vi "SP_OEE_2_test.vi"() -> ()   [LabVIEW 2017]
uses:
  <vilib>/addons/database/Connection.llb/DB Tools Open Connec (Path).vi
  <vilib>/addons/database/_DB Variant To Data/Database Variant To Data.xnode
  <vilib>/addons/database/NI_Database_API.lvlib
panel:
  in  "Left Button":bool
  in  "Report Button":bool
  out "Array":string[][](array[string])
  out "OEE":dbl format="%#_4g"
  out "IDEAL CYCLE TIME":i32
  out "CAPACITY":dbl
  out "AVAILABLILITY TIME(MIN)":i32
  out "PERFORMANCE":dbl format="%#_4g"
  out "QUALITY":dbl format="%#_4g"
  out "Production count":i32
  out "transposed array":string[][](array[string])
  out "CYCLE TIME":string[](array[string])
  out "ACTUAL PROD TIME":string[](array[string])
  out "?":string[][](array[string])
  out "error out":errorcluster
  in  "wise":string(combo)
  out "Date Count":string[](array[string])
  out "Sorted Date":string[](array[string])
  out "ALL DATE":string[](array[string])
  in  "error in (no error)":errorcluster
  in  "Download":bool
  in  "Shift":string(combo)
  in  "Tab Control":enum32{"Statistical", "Graphical"}(tab)
  out "Table":string[][](table)
  out "Table 2":string[][](table)
  out "Run-Time Status":cluster{"Array 2":timestamp[], dbl[]}(graph)
  in  "Select Station":string(combo)
  in  "To Date":timestamp format="%<%Y-%m-%d>T"
  in  "Form Date":timestamp format="%<%Y-%m-%d>T"
  in  "Select Stakeholder":string(combo)
  # "OEE REPORT"
  # "%"
  # "Date"
  # "Safety"
  # "Logistic"
  # "Maintenance"
  # "Quality"
  # "Production"
  # "Total"
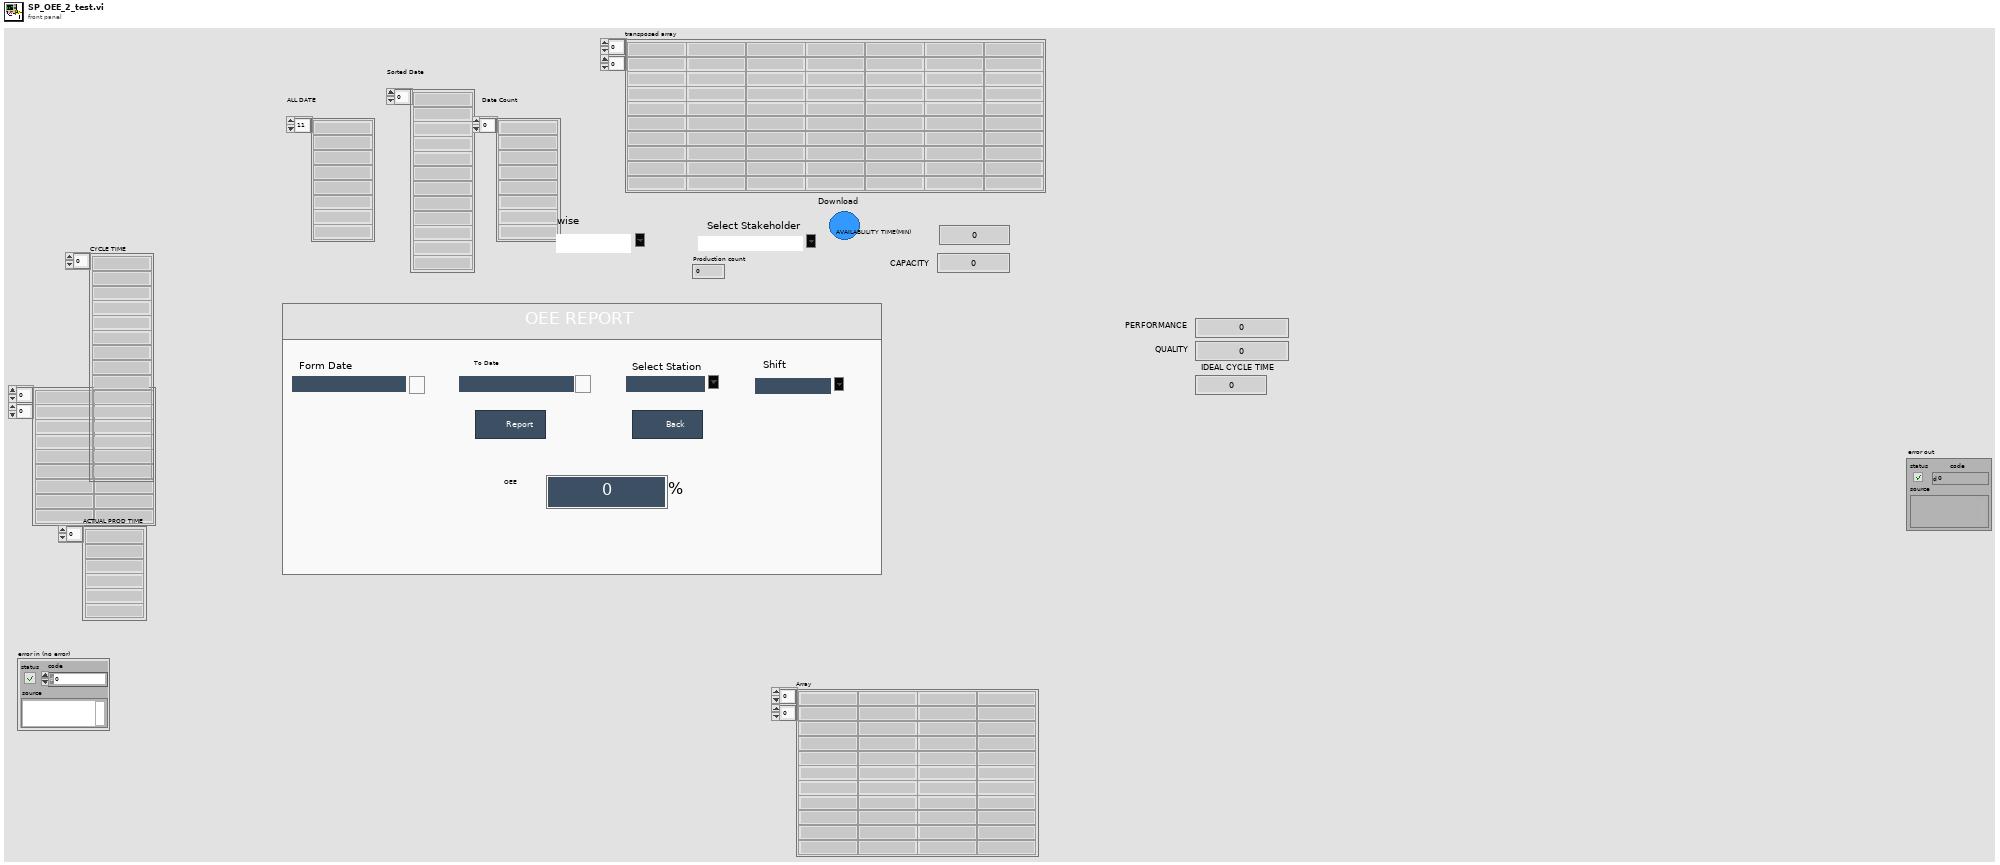
[diagram p1: front panel]
types:
  T1 = typedef "LVDateTimeRec.ctl" = cluster{"fractional second":dbl, "second":i32, "minute":i32, "hour":i32, "day of month":i32, "month":i32, "year":i32, "day of week":i32, "day of year":i32, "DST":i32}
  T2 = typedef "NI_Database_API.lvlib/Conn ObjectReference.ctl" = refnum<k1>
  T3 = enum32{"invalid app kind", "Development System", "Run Time System", "Student Edition", "Embedded LabVIEW", "Evaluation", "Custom"}
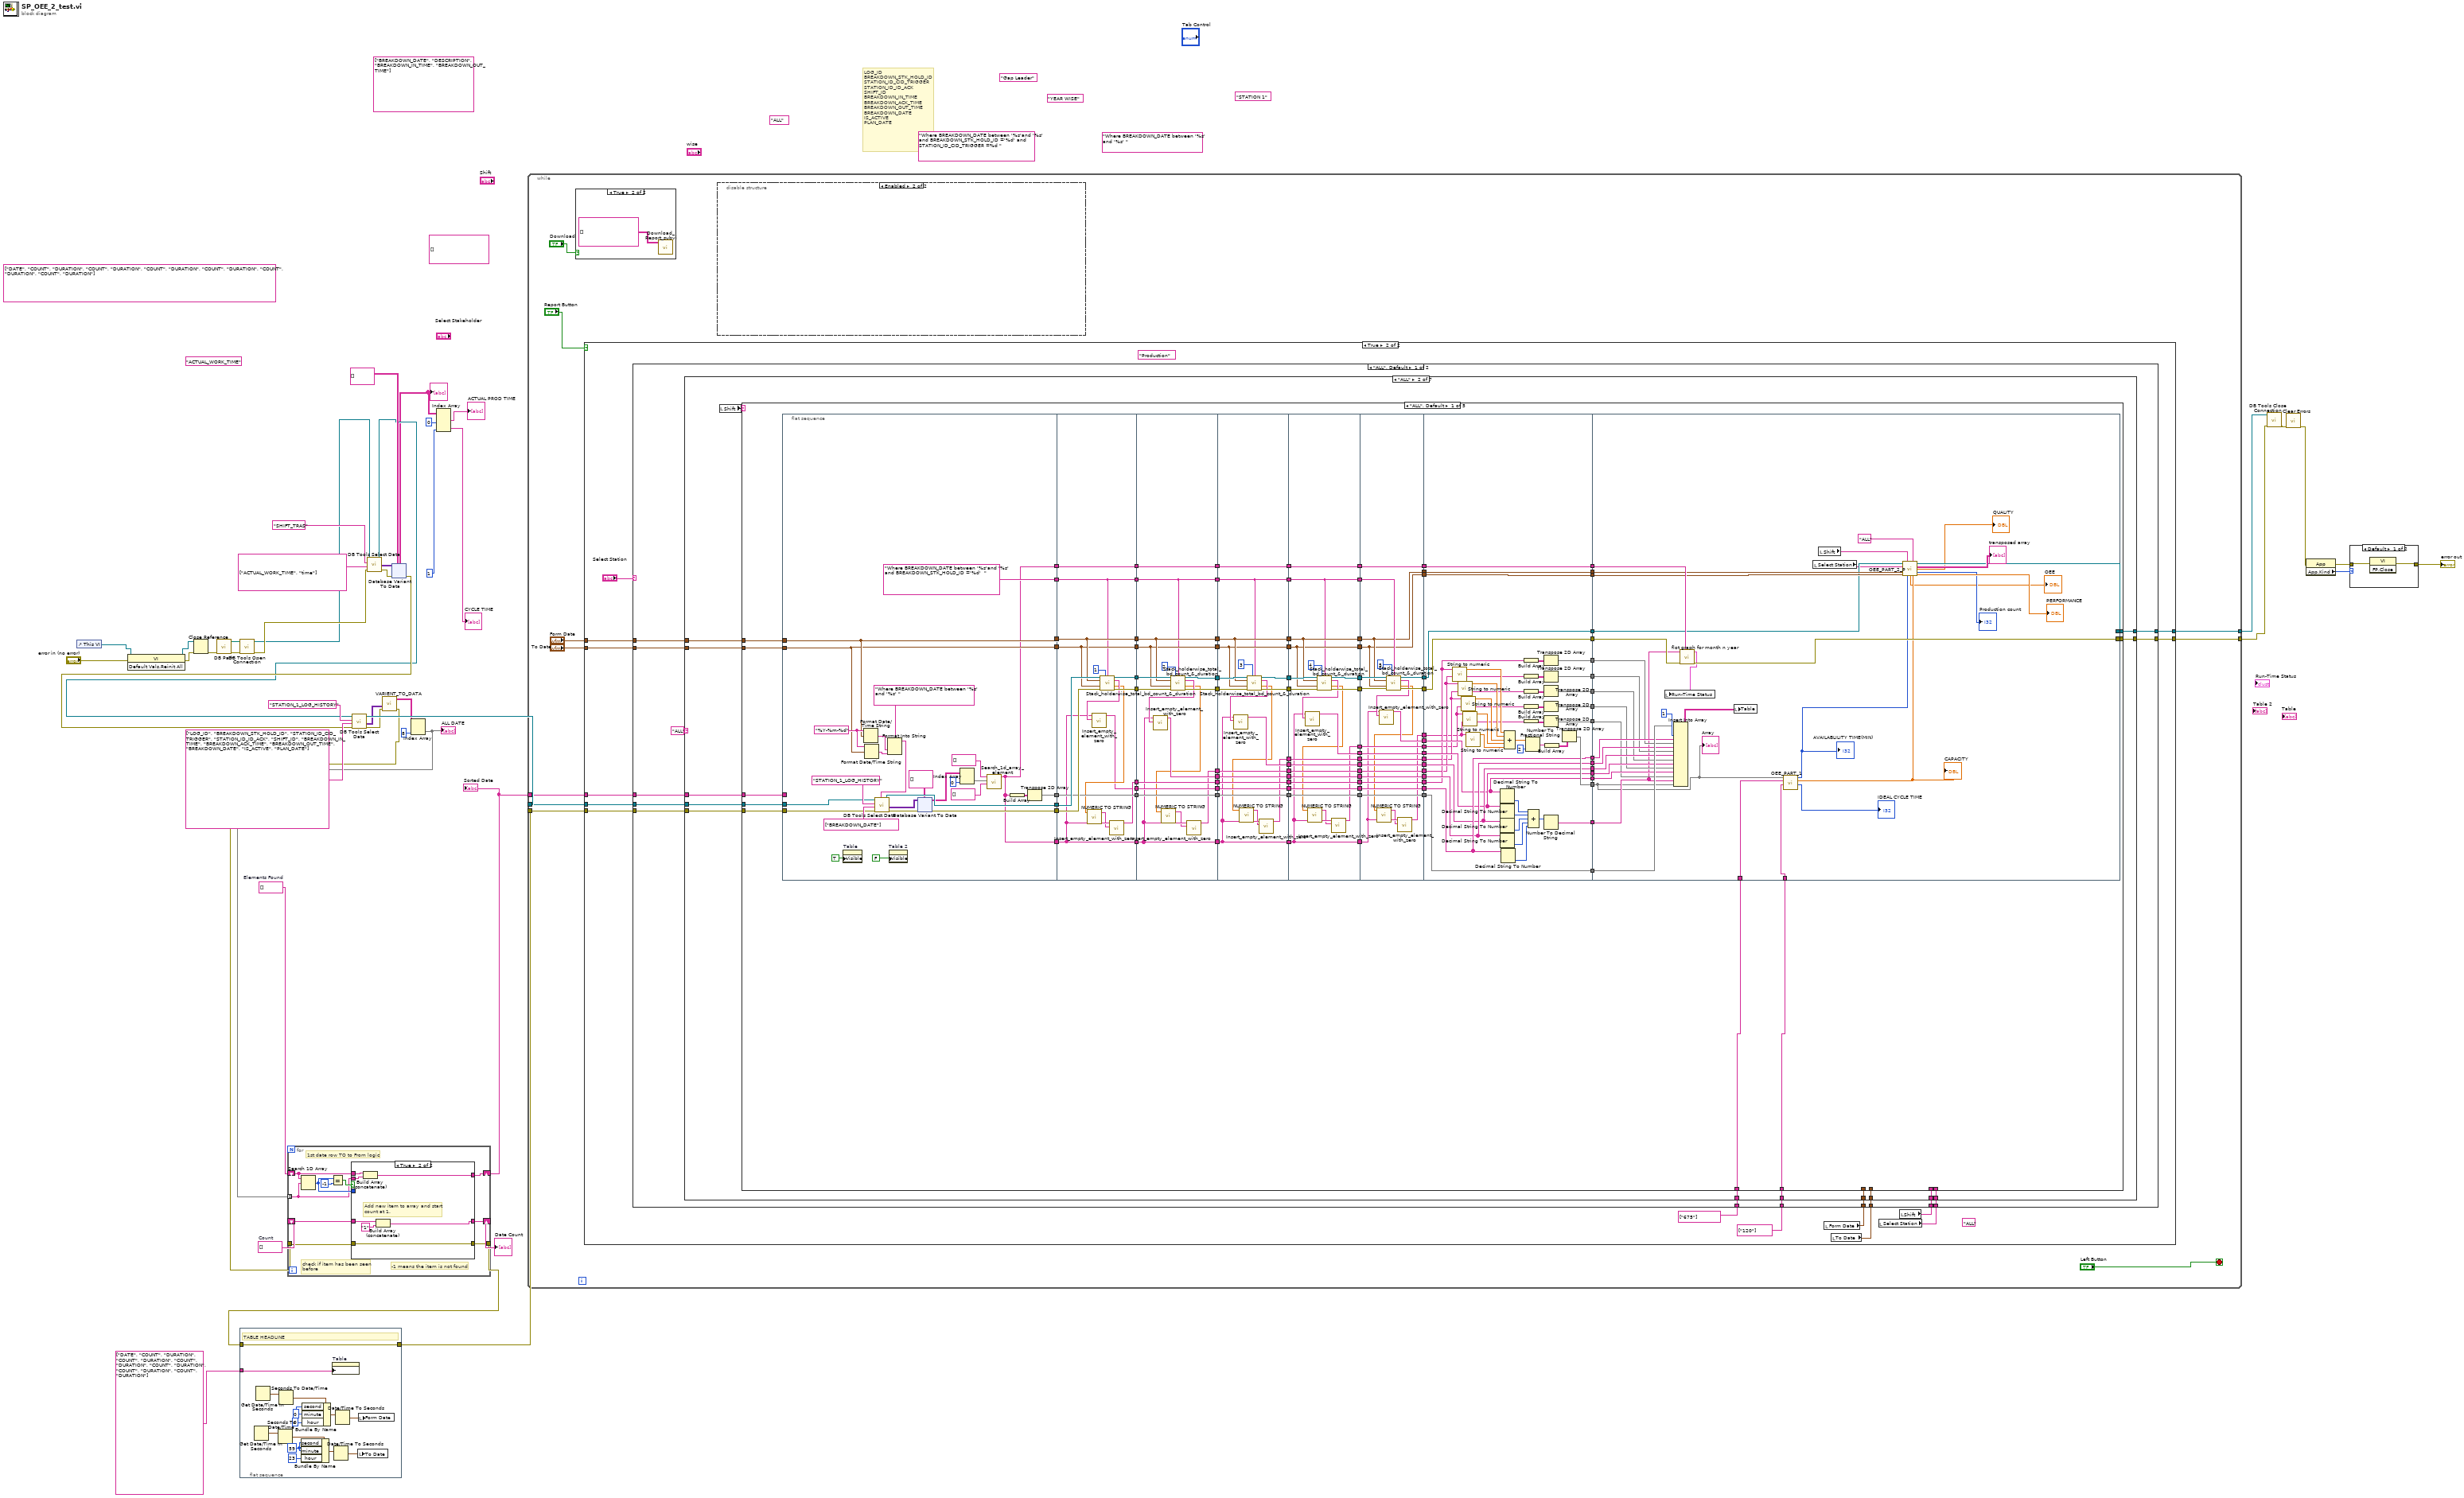
[diagram p0: block diagram]
diagram:
  (unwired) string[][] [] ("Column Header Strings[]")
  (unwired) string[][] [["DATE", "COUNT", "DURATION", "COUNT", "DURATION", "COUNT", "DURATION", "COUNT", "DURATION", "COUNT", "DURATION", "COUNT", "DURATION"]] ("Column Header Strings[]")
  (unwired) "ACTUAL_WORK_TIME" ("String")
  (unwired) "Where BREAKDOWN_DATE between '%s' and '%s' "
  (unwired) "Where BREAKDOWN_DATE between '%s'and '%s' and BREAKDOWN_STK_HOLD_ID ='%d' and STATION_ID_CID_TRIGGER =%d "
  (unwired) "ALL" ("Shift")
  (unwired) "STATION 1" ("Select Station")
  (unwired) "Gap Leader" ("Select Stakeholder")
  (unwired) string[] ["BREAKDOWN_DATE", "DESCRIPTION", "BREAKDOWN_IN_TIME", "BREAKDOWN_OUT_TIME"]
  (unwired) "YEAR WISE" ("wise")
  w34 = string[] []  # Count
  w35 = string[] []  # Elements Found
  # "LOG_ID\nBREAKDOWN_STK_HOLD_ID\nSTATION_ID_CID_TRIGGER\nSTATION_ID_ID_ACK\nSHIFT_ID\nBREAKDOWN_IN_TIME\nBREAKDOWN_ACK_TIME\nBREAKDOWN_OUT_TIME\nBREAKDOWN_DATE\nIS_ACTIVE\nPLAN_DATE"
  n1 = control-ref of="This VI"() -> (w44:refnum<vi>)
  n2 = invoke class="VI" method="Default Vals.Reinit All"(reference=w44, error in="error in (no error)") -> (reference out=w42:refnum<vi>, error out=w43:errorcluster)  [unwired: 1 in, 1 out]
  n3 = Close Reference(reference=w42, error in (no error)=w43) -> (error out=w41:errorcluster)
  n4 = call "DB Path.vi"("error in"=w41) -> ("error out"=w40:errorcluster, "DB Path"=w39:path)  [unwired: 9 in]
  n5 = flat-sequence {
    tunnel: [w58] -> w27
    tunnel: w30 -> [w58]
    tunnel: string[] ["DATE", "COUNT", "DURATION", "COUNT", "DURATION", "COUNT", "DURATION", "COUNT", "DURATION", "COUNT", "DURATION", "COUNT", "DURATION"] ("Column Header Strings[]") -> [w45]
    frame #0 {
      w48 = 59 ("second")
      w54 = 0 ("second")
      # "TABLE HEADLINE"
      n6 = Get Date/Time In Seconds() -> (seconds since 1Jan1904=w51:timestamp)
      n7 = Get Date/Time In Seconds() -> (seconds since 1Jan1904=w55:timestamp)
      n8 = Seconds To Date/Time(time stamp (now)=w51) -> (date time rec=w50:T1)  [unwired: 1 in]
      n9 = Seconds To Date/Time(time stamp (now)=w55) -> (date time rec=w56:T1)  [unwired: 1 in]
      n10 = Bundle By Name(cluster=w50, "second"=w48, "minute"=w48, "hour"=23) -> (w49:T1)
      n11 = Bundle By Name(cluster=w56, "second"=w54, "minute"=w54, "hour"=0) -> (w57:T1)
      n12 = property on="Table" class="Tbl (strict)"("Column Headers[]"=w45) -> ()  [unwired: 2 in, 2 out]
      n13 = Date/Time To Seconds(2:w49) -> (0:w46:timestamp)  [unwired: 1 in]
      n14 = Date/Time To Seconds(2:w57) -> (0:w52:timestamp)  [unwired: 1 in]
      n15 = local write "To Date"(w46) -> ()
      n16 = local write "Form Date"(w52) -> ()
    }
  }
  n17 = call-poly <vilib>:"DB Tools Open Connection.vi"("error in (no error)"=w40, "connection information"=w39) -> ("error out"=w9:errorcluster, "connection reference"=w7:T2)  [unwired: 6 in]
  n18 = call <vilib>:"DB Tools Select Data.vi"("error in (no error)"=w9, "columns"=string[] ["ACTUAL_WORK_TIME", "time"], "table"="SHIFT_TRAS", "connection reference"=w7) -> ("error out"=w13:errorcluster, "data"=w12:variant[][], "connection reference out"=w6:T2)  [unwired: 2 in]
  n19 = xnode "Database Variant To Data"("database variant"=w12, "error in (no error)"=w13, "type"=string[][] []) -> ("data"=w5:string[][], "error out"=w10:errorcluster)
  "?" <- w5
  n20 = call <vilib>:"DB Tools Select Data.vi"("error in (no error)"=w10, "columns"=string[] ["LOG_ID", "BREAKDOWN_STK_HOLD_ID", "STATION_ID_CID_TRIGGER", "STATION_ID_ID_ACK", "SHIFT_ID", "BREAKDOWN_IN_TIME", "BREAKDOWN_ACK_TIME", "BREAKDOWN_OUT_TIME", "BREAKDOWN_DATE", "IS_ACTIVE", "PLAN_DATE"], "table"="STATION_1_LOG_HISTORY", "connection reference"=w6) -> ("error out"=w24:errorcluster, "data"=w25:variant[][], "connection reference out"=w29:T2)  [unwired: 2 in]
  n21 = call "VARIENT_TO_DATA.vi"("data"=w25, "error in (no error)"=w24) -> ("Table"=w22:string[][], "error out"=w23:errorcluster)  [unwired: 7 in]
  n22 = Index Array(array=w22, index (col)=8 ("disabled index (col)")) -> (element=w33:string[])  [unwired: 1 in]
  "ALL DATE" <- w33
  n23 = for {
    tunnel: w33 -> [w61] mode=indexing
    shift-right: [w65] -> w26
    shift-left: w35 -> [w66]
    shift-right: [w63] -> w32
    shift-left: w34 -> [w64]
    tunnel: [w60] -> w30
    tunnel: w23 -> [w59]
    # "1st date row TO to From logic"
    # "-1 means the item is not found"
    # "check if item has been seen\nbefore"
    n24 = Search 1D Array(1D array=w66, element=w61) -> (index of element=w62:i32)  [unwired: 1 in]
    n25 = Equal?(x=w62, y=-1) -> (x = y?=w67:bool)
    n26 = case shown="True" w67 {
      tunnel: w66 -> [w77 w84]
      tunnel: [w77 w83] -> w65
      tunnel: w64 -> [w76 w82]
      tunnel: [w74 w81] -> w63
      tunnel: w62 -> [w75 _]
      tunnel: w61 -> [_ w79]
      tunnel: [w69 w78] -> w60
      tunnel: w59 -> [w69 w78]
      frame False {
        # "Item has been Seen before,\nincrement count"
        n27 = Index Array(array=w76, index=w75) -> (element=w73:string)
        n28 = Decimal String To Number(string=w73) -> (number=w72:i32)  [unwired: 2 in, 1 out]
        n29 = Increment(x=w72) -> (x+1=w71:i32)
        n30 = Number To Decimal String(number=w71) -> (decimal integer string=w70:string)  [unwired: 1 in]
        n31 = Replace Array Subset(array=w76, new element=w70, index=w75) -> (w74:string[])
      }
      frame True {
        # "Add new item to array and start\ncount at 1."
        n32 = Build Array (concatenate)(w84, w79) -> (w83:string[])
        n33 = Build Array (concatenate)(w82, "1") -> (w81:string[])
      }
    }
  }
  "Sorted Date" <- w26
  "Date Count" <- w32
  n34 = Index Array(array=w5, index (col) #1=0 ("disabled index (col)"), index (col) #2=1 ("disabled index (col)")) -> (element #1=→"ACTUAL PROD TIME":string[], element #2=→"CYCLE TIME":string[])  [unwired: 2 in]
  n35 = while {
    tunnel: w29 -> [w94]
    tunnel: w27 -> [w93]
    tunnel: w26 -> [w92]
    tunnel: [w89] -> w16
    tunnel: [w88] -> w15
    stop <- "Left Button" stop-if-true
    n36 = case shown="True" "Download" {
      frame False {
      }
      frame True {
        n37 = call "Download_Report_subvi.vi"("Column Header Strings[]"=string[][] []) -> ()  [unwired: 10 in, 1 out]
      }
    }
    n38 = case shown="True" "Report Button" {
      tunnel: w94 -> [_ w164]
      tunnel: w93 -> [_ w163]
      tunnel: w92 -> [_ w162]
      tunnel: "Form Date" -> [_ w161]
      tunnel: "To Date" -> [_ w160]
      tunnel: [_ w158] -> w89
      tunnel: [_ w157] -> w88
      frame False {
      }
      frame True {
        (unwired) "ALL" ("String")
        (unwired) "Production" ("Select\n Stakeholder")
        n39 = local read "Form Date"() -> (w156:timestamp)
        n40 = local read "To Date"() -> (w155:timestamp)
        n41 = local read "Select Station"() -> (w153:string)
        n42 = local read "Shift"() -> (w154:string)
        n43 = case shown="\"ALL\", Default" "Select Station" {
          tunnel: w164 -> [w178 w9178]
          tunnel: w163 -> [w177 w9177]
          tunnel: w162 -> [w176 w9176]
          tunnel: w161 -> [w175 w9175]
          tunnel: w160 -> [w174 w9174]
          tunnel: [w172 w9173] -> w158
          tunnel: [w171 w9172] -> w157
          tunnel: string[] ["675"] -> [w170 w9168]
          tunnel: string[] ["120"] -> [w169 w9167]
          tunnel: w156 -> [w168 w9170]
          tunnel: w155 -> [w167 w9169]
          tunnel: w154 -> [w166 w9166]
          tunnel: w153 -> [w165 w9165]
          frame "ALL", Default {
            n44 = case shown="\"ALL\"" "ALL" {
              tunnel: w178 -> [_ w192 w1621 w3106 w4604 w6111 w7633]
              tunnel: w177 -> [_ w191 w1620 w3105 w4603 w6110 w7632]
              tunnel: w176 -> [_ w190 w1619 w3104 w4602 w6109 w7631]
              tunnel: w175 -> [_ w189 w1618 w3103 w4601 w6108 w7630]
              tunnel: w174 -> [_ w188 w1617 w3102 w4600 w6107 w7629]
              tunnel: [_ w186 w1615 w3100 _ _ _] -> w172
              tunnel: [_ w185 w1614 w3099 _ _ _] -> w171
              tunnel: w170 -> [_ w184 _ _ _ _ _]
              tunnel: w169 -> [_ w183 _ _ _ _ _]
              tunnel: w168 -> [_ w182 _ _ _ _ _]
              tunnel: w167 -> [_ w181 _ _ _ _ _]
              tunnel: w166 -> [_ w180 _ _ _ _ _]
              tunnel: w165 -> [_ w179 _ _ _ _ _]
              frame "False", Default {
              }
              frame "ALL" {
                n45 = local read "Shift"() -> (w187:string)
                n46 = case shown="\"ALL\", Default" w187 {
                  selector: w187 -> [_ w563 w919 w1275 _]
                  tunnel: w192 -> [w205 w572 w928 w1284 _]
                  tunnel: w191 -> [w204 w571 w927 w1283 _]
                  tunnel: w190 -> [w203 w570 w926 w1282 _]
                  tunnel: w189 -> [w194 w569 w925 w1281 _]
                  tunnel: w188 -> [w193 w568 w924 w1280 _]
                  tunnel: [w202 w546 w902 w1258 _] -> w186
                  tunnel: [w201 w547 w903 w1259 _] -> w185
                  tunnel: w184 -> [w200 w562 w918 w1273 _]
                  tunnel: w183 -> [w199 w561 w917 w1272 _]
                  tunnel: w182 -> [_ w559 w915 w1270 _]
                  tunnel: w181 -> [_ w558 w914 w1269 _]
                  tunnel: w180 -> [_ w557 w913 w1267 _]
                  tunnel: w179 -> [_ w556 w911 w1268 _]
                  frame "ALL", Default {
                    n47 = flat-sequence {
                      tunnel: w205 -> [w317]
                      tunnel: w204 -> [w315]
                      tunnel: [w301] -> w295
                      tunnel: [w316] -> w294
                      tunnel: w203 -> [_]
                      tunnel: [w320] -> w293
                      tunnel: [w300] -> w292
                      tunnel: [w299] -> w291
                      tunnel: [w297] -> w290
                      tunnel: w194 -> [w300]
                      tunnel: w193 -> [w299]
                      tunnel: ["Where BREAKDOWN_DATE between '%s'and '%s' and BREAKDOWN_STK_HOLD_ID ='%d'  "] -> w289
                      tunnel: [w297] -> w288
                      tunnel: w295 -> [w380]
                      tunnel: w294 -> [w382]
                      tunnel: w293 -> [w377]
                      tunnel: w292 -> [w376]
                      tunnel: w291 -> [w375]
                      tunnel: [w379] -> w287
                      tunnel: [w381] -> w286
                      tunnel: [w377] -> w285
                      tunnel: [w367] -> w284
                      tunnel: [w373] -> w283
                      tunnel: [w376] -> w282
                      tunnel: [w375] -> w281
                      tunnel: w290 -> [w372]
                      tunnel: [w372] -> w280
                      tunnel: w289 -> [w369]
                      tunnel: [w369] -> w279
                      tunnel: [w368] -> w278
                      tunnel: w288 -> [w368]
                      tunnel: w287 -> [w397]
                      tunnel: w286 -> [w395]
                      tunnel: w285 -> [w400]
                      tunnel: w284 -> [w399]
                      tunnel: w283 -> [w398]
                      tunnel: w282 -> [w392]
                      tunnel: w281 -> [w391]
                      tunnel: [w400] -> w277
                      tunnel: [w399] -> w276
                      tunnel: [w398] -> w275
                      tunnel: [w396] -> w274
                      tunnel: [w389] -> w273
                      tunnel: [w388] -> w272
                      tunnel: [w393] -> w271
                      tunnel: [w392] -> w270
                      tunnel: [w391] -> w269
                      tunnel: w280 -> [w387]
                      tunnel: [w387] -> w268
                      tunnel: w279 -> [w384]
                      tunnel: [w384] -> w267
                      tunnel: [w383] -> w266
                      tunnel: w278 -> [w383]
                      tunnel: w277 -> [w420]
                      tunnel: w276 -> [w419]
                      tunnel: w275 -> [w418]
                      tunnel: w274 -> [w414]
                      tunnel: w273 -> [w417]
                      tunnel: w272 -> [w416]
                      tunnel: w271 -> [w412]
                      tunnel: w270 -> [w410]
                      tunnel: w269 -> [w409]
                      tunnel: [w420] -> w265
                      tunnel: [w419] -> w264
                      tunnel: [w418] -> w263
                      tunnel: [w417] -> w262
                      tunnel: [w416] -> w261
                      tunnel: [w413] -> w260
                      tunnel: [w407] -> w259
                      tunnel: [w406] -> w258
                      tunnel: [w411] -> w257
                      tunnel: [w410] -> w256
                      tunnel: [w409] -> w255
                      tunnel: w268 -> [w405]
                      tunnel: [w405] -> w254
                      tunnel: w267 -> [w402]
                      tunnel: [w402] -> w253
                      tunnel: [w401] -> w252
                      tunnel: w266 -> [w401]
                      tunnel: w265 -> [w442]
                      tunnel: w264 -> [w441]
                      tunnel: w263 -> [w440]
                      tunnel: w262 -> [w439]
                      tunnel: w261 -> [w438]
                      tunnel: w260 -> [w434]
                      tunnel: w259 -> [w437]
                      tunnel: w258 -> [w436]
                      tunnel: w257 -> [w433]
                      tunnel: w256 -> [w430]
                      tunnel: w255 -> [w429]
                      tunnel: [w442] -> w251
                      tunnel: [w441] -> w250
                      tunnel: [w440] -> w249
                      tunnel: [w439] -> w248
                      tunnel: [w438] -> w247
                      tunnel: [w437] -> w246
                      tunnel: [w436] -> w245
                      tunnel: [w432] -> w244
                      tunnel: [w431] -> w243
                      tunnel: [w427] -> w242
                      tunnel: [w426] -> w241
                      tunnel: [w430] -> w240
                      tunnel: [w429] -> w239
                      tunnel: w254 -> [w425]
                      tunnel: [w425] -> w238
                      tunnel: w253 -> [w422]
                      tunnel: [w422] -> w237
                      tunnel: [w421] -> w236
                      tunnel: w252 -> [w421]
                      tunnel: w251 -> [w466]
                      tunnel: w250 -> [w465]
                      tunnel: w249 -> [w464]
                      tunnel: w248 -> [w463]
                      tunnel: w247 -> [w462]
                      tunnel: w246 -> [w461]
                      tunnel: w245 -> [w460]
                      tunnel: w244 -> [w454]
                      tunnel: w243 -> [w456]
                      tunnel: w242 -> [w459]
                      tunnel: w241 -> [w458]
                      tunnel: w240 -> [w444]
                      tunnel: w239 -> [w443]
                      tunnel: [w466] -> w235
                      tunnel: [w465] -> w234
                      tunnel: [w464] -> w233
                      tunnel: [w463] -> w232
                      tunnel: [w462] -> w231
                      tunnel: [w461] -> w230
                      tunnel: [w460] -> w229
                      tunnel: [w459] -> w228
                      tunnel: [w458] -> w227
                      tunnel: [w455] -> w226
                      tunnel: [w453] -> w225
                      tunnel: [w451] -> w224
                      tunnel: [w449] -> w223
                      tunnel: w238 -> [w450]
                      tunnel: w237 -> [w446]
                      tunnel: [w445] -> w222
                      tunnel: w236 -> [w445]
                      tunnel: [w444] -> w197
                      tunnel: [w443] -> w195
                      tunnel: w235 -> [w495]
                      tunnel: w234 -> [w488]
                      tunnel: w233 -> [w479]
                      tunnel: w232 -> [w487]
                      tunnel: w231 -> [w477]
                      tunnel: w230 -> [w486]
                      tunnel: w229 -> [w475]
                      tunnel: w228 -> [w485]
                      tunnel: w227 -> [w473]
                      tunnel: w226 -> [w509]
                      tunnel: w225 -> [w508]
                      tunnel: w224 -> [w484]
                      tunnel: w223 -> [w471]
                      tunnel: [w509] -> w221
                      tunnel: [w508] -> w220
                      tunnel: [w502] -> w219
                      tunnel: [w495] -> w218
                      tunnel: [w494] -> w217
                      tunnel: [w493] -> w216
                      tunnel: [w492] -> w215
                      tunnel: [w491] -> w214
                      tunnel: [w490] -> w213
                      tunnel: [w489] -> w212
                      tunnel: [w488] -> w211
                      tunnel: [w487] -> w210
                      tunnel: [w486] -> w209
                      tunnel: [w485] -> w208
                      tunnel: [w484] -> w207
                      tunnel: [w469] -> w206
                      tunnel: w222 -> [w469]
                      tunnel: [w468] -> w198
                      tunnel: w197 -> [w468]
                      tunnel: [w467] -> w196
                      tunnel: w195 -> [w467]
                      tunnel: [w518] -> w201
                      tunnel: [w532] -> w202
                      tunnel: w221 -> [w533]
                      tunnel: w220 -> [w519]
                      tunnel: w219 -> [w531]
                      tunnel: w218 -> [w544]
                      tunnel: w217 -> [w542]
                      tunnel: w216 -> [w540]
                      tunnel: w215 -> [w538]
                      tunnel: w214 -> [w536]
                      tunnel: w213 -> [w534]
                      tunnel: w212 -> [w527]
                      tunnel: w211 -> [w543]
                      tunnel: w210 -> [w541]
                      tunnel: w209 -> [w539]
                      tunnel: w208 -> [w537]
                      tunnel: w207 -> [w535]
                      tunnel: w206 -> [w530]
                      tunnel: w200 -> [w526]
                      tunnel: w199 -> [w525]
                      tunnel: w198 -> [w523]
                      tunnel: w196 -> [w522]
                      frame #0 {
                        w308 = "%Y-%m-%d" ("time format string (%c)")
                        n48 = property on="Table" class="Tbl (strict)"("Visible"=TRUE) -> ()  [unwired: 2 in, 2 out]
                        n49 = Format Date/Time String(time format string (%c)=w308, seconds (now)=w300) -> (date/time string=w309:string)  [unwired: 1 in]
                        n50 = Format Date/Time String(time format string (%c)=w308, seconds (now)=w299) -> (date/time string=w307:string)  [unwired: 1 in]
                        n51 = Format Into String(format string="Where BREAKDOWN_DATE between '%s' and '%s' ", w309, w307) -> (resulting string=w306:string)  [unwired: 2 in, 1 out]
                        n52 = call <vilib>:"DB Tools Select Data.vi"("condition"=w306, "error in (no error)"=w315, "columns"=string[] ["BREAKDOWN_DATE"], "table"="STATION_1_LOG_HISTORY", "connection reference"=w317) -> ("error out"=w302:errorcluster, "data"=w305:variant[][], "connection reference out"=w316:T2)  [unwired: 1 in]
                        n53 = property on="Table 2" class="Tbl (strict)"("Visible"=FALSE) -> ()  [unwired: 2 in, 2 out]
                        n54 = xnode "Database Variant To Data"("database variant"=w305, "error in (no error)"=w302, "type"=string[][] [] ("Elements Found")) -> ("data"=w303:string[][], "error out"=w301:errorcluster)
                        n55 = Index Array(array=w303, index (col)=0 ("disabled index (col)")) -> (element=w311:string[])  [unwired: 1 in]
                        n56 = call "Search_1d_array_element.vi"("Count in"=string[] [] ("Elements Found"), "BD Date"=w311, "Elements Found in"=string[] [] ("Elements Found")) -> ("Elements Found out"=w297:string[])  [unwired: 4 in, 2 out]
                        n57 = Build Array(w297) -> (w321:string[][])
                        n58 = Transpose 2D Array(2D array=w321) -> (transposed array=w320:string[][])
                      }
                      frame #1 {
                        n59 = call "Stack_holderwise_total_bd_count_&_duration.vi"("Refnum in"=w382, "BREAKDOWN_STK_HOLD_ID"=1, "condition"=w369, "Form Date"=w376, "To Date"=w375, "error in (no error)"=w380) -> ("Refnum out"=w381:T2, "Count out"=w374:string[], "appended array"=w371:dbl[], "error out"=w379:errorcluster)  [unwired: 6 in]
                        n60 = call "NUMERIC TO STRING.vi"("appended array"=w371) -> ("Array"=w370:string[])  [unwired: 4 in]
                        n61 = call "Insert_empty_element_with_zero.vi"("searched date"=w374, "fixed date"=w372) -> ("O/P"=w367:string[])  [unwired: 9 in]
                        n62 = call "Insert_empty_element_with_zero.vi"("searched date"=w370, "fixed date"=w372) -> ("O/P"=w373:string[])  [unwired: 9 in]
                      }
                      frame #2 {
                        n63 = call "Stack_holderwise_total_bd_count_&_duration.vi"("Refnum in"=w395, "BREAKDOWN_STK_HOLD_ID"=2, "condition"=w384, "Form Date"=w392, "To Date"=w391, "error in (no error)"=w397) -> ("Refnum out"=w393:T2, "Count out"=w390:string[], "appended array"=w386:dbl[], "error out"=w396:errorcluster)  [unwired: 6 in]
                        n64 = call "Insert_empty_element_with_zero.vi"("searched date"=w390, "fixed date"=w387) -> ("O/P"=w389:string[])  [unwired: 9 in]
                        n65 = call "NUMERIC TO STRING.vi"("appended array"=w386) -> ("Array"=w385:string[])  [unwired: 4 in]
                        n66 = call "Insert_empty_element_with_zero.vi"("searched date"=w385, "fixed date"=w387) -> ("O/P"=w388:string[])  [unwired: 9 in]
                      }
                      frame #3 {
                        n67 = call "Stack_holderwise_total_bd_count_&_duration.vi"("Refnum in"=w412, "BREAKDOWN_STK_HOLD_ID"=3, "condition"=w402, "Form Date"=w410, "To Date"=w409, "error in (no error)"=w414) -> ("Refnum out"=w411:T2, "Count out"=w408:string[], "appended array"=w404:dbl[], "error out"=w413:errorcluster)  [unwired: 6 in]
                        n68 = call "Insert_empty_element_with_zero.vi"("searched date"=w408, "fixed date"=w405) -> ("O/P"=w407:string[])  [unwired: 9 in]
                        n69 = call "NUMERIC TO STRING.vi"("appended array"=w404) -> ("Array"=w403:string[])  [unwired: 4 in]
                        n70 = call "Insert_empty_element_with_zero.vi"("searched date"=w403, "fixed date"=w405) -> ("O/P"=w406:string[])  [unwired: 9 in]
                      }
                      frame #4 {
                        n71 = call "Stack_holderwise_total_bd_count_&_duration.vi"("Refnum in"=w433, "BREAKDOWN_STK_HOLD_ID"=4, "condition"=w422, "Form Date"=w430, "To Date"=w429, "error in (no error)"=w434) -> ("Refnum out"=w432:T2, "Count out"=w428:string[], "appended array"=w424:dbl[], "error out"=w431:errorcluster)  [unwired: 6 in]
                        n72 = call "Insert_empty_element_with_zero.vi"("searched date"=w428, "fixed date"=w425) -> ("O/P"=w427:string[])  [unwired: 9 in]
                        n73 = call "NUMERIC TO STRING.vi"("appended array"=w424) -> ("Array"=w423:string[])  [unwired: 4 in]
                        n74 = call "Insert_empty_element_with_zero.vi"("searched date"=w423, "fixed date"=w425) -> ("O/P"=w426:string[])  [unwired: 9 in]
                      }
                      frame #5 {
                        n75 = call "Stack_holderwise_total_bd_count_&_duration.vi"("Refnum in"=w454, "BREAKDOWN_STK_HOLD_ID"=5, "condition"=w446, "Form Date"=w444, "To Date"=w443, "error in (no error)"=w456) -> ("Refnum out"=w453:T2, "Count out"=w452:string[], "appended array"=w448:dbl[], "error out"=w455:errorcluster)  [unwired: 6 in]
                        n76 = call "NUMERIC TO STRING.vi"("appended array"=w448) -> ("Array"=w447:string[])  [unwired: 4 in]
                        n77 = call "Insert_empty_element_with_zero.vi"("searched date"=w452, "fixed date"=w450) -> ("O/P"=w451:string[])  [unwired: 9 in]
                        n78 = call "Insert_empty_element_with_zero.vi"("searched date"=w447, "fixed date"=w450) -> ("O/P"=w449:string[])  [unwired: 9 in]
                      }
                      frame #6 {
                        n79 = call "String to numeric.vi"("Array"=w479) -> ("Array 2"=w478:dbl[])  [unwired: 4 in]
                        n80 = call "String to numeric.vi"("Array"=w477) -> ("Array 2"=w476:dbl[])  [unwired: 4 in]
                        n81 = call "String to numeric.vi"("Array"=w475) -> ("Array 2"=w474:dbl[])  [unwired: 4 in]
                        n82 = call "String to numeric.vi"("Array"=w473) -> ("Array 2"=w472:dbl[])  [unwired: 4 in]
                        n83 = call "String to numeric.vi"("Array"=w471) -> ("Array 2"=w470:dbl[])  [unwired: 4 in]
                        n84 = Decimal String To Number(string=w484) -> (number=w503:i32[])  [unwired: 2 in, 1 out]
                        n85 = Decimal String To Number(string=w485) -> (number=w504:i32[])  [unwired: 2 in, 1 out]
                        n86 = Decimal String To Number(string=w486) -> (number=w505:i32[])  [unwired: 2 in, 1 out]
                        n87 = Decimal String To Number(string=w487) -> (number=w506:i32[])  [unwired: 2 in, 1 out]
                        n88 = Decimal String To Number(string=w488) -> (number=w501:i32[])  [unwired: 2 in, 1 out]
                        n89 = Compound Arithmetic op=ADD(w478, w476, w474, w472, w470) -> (w481:dbl[])
                        n90 = Build Array(w479) -> (w500:string[][])
                        n91 = Build Array(w477) -> (w499:string[][])
                        n92 = Build Array(w475) -> (w498:string[][])
                        n93 = Build Array(w473) -> (w497:string[][])
                        n94 = Build Array(w471) -> (w496:string[][])
                        n95 = Number To Fractional String(number=w481, precision (6)=i16 2) -> (F-format string=w480:string[])  [unwired: 2 in]
                        n96 = Compound Arithmetic op=ADD(w503, w504, w505, w506, w501) -> (w507:i32[])
                        n97 = Transpose 2D Array(2D array=w500) -> (transposed array=w494:string[][])
                        n98 = Transpose 2D Array(2D array=w499) -> (transposed array=w493:string[][])
                        n99 = Transpose 2D Array(2D array=w498) -> (transposed array=w492:string[][])
                        n100 = Transpose 2D Array(2D array=w497) -> (transposed array=w491:string[][])
                        n101 = Transpose 2D Array(2D array=w496) -> (transposed array=w490:string[][])
                        n102 = Number To Decimal String(number=w507) -> (decimal integer string=w502:string[])  [unwired: 1 in]
                        n103 = Build Array(w480) -> (w483:string[][])
                        n104 = Transpose 2D Array(2D array=w483) -> (transposed array=w489:string[][])
                      }
                      frame #7 {
                        n105 = Insert Into Array(array=w544, index (col)=1 ("disabled index (col)"), new element #1=w543, new element #2=w542, new element #3=w541, new element #4=w540, new element #5=w539, new element #6=w538, new element #7=w537, new element #8=w536, new element #9=w535, new element #10=w534, new element #11=w531, new element #12=w527) -> (w529:string[][])  [unwired: 1 in]
                        n106 = call "flot graph for month n year.vi"("BD Date"=w530, "error in (no error)"=w533, "Count total"=w531) -> ("error out"=w532:errorcluster, "Run-Time Status"=w528:cluster{"Array 2":timestamp[], dbl[]})  [unwired: 7 in]
                        n107 = local write "Run-Time Status"(w528) -> ()
                        n108 = local write "Table"(w529) -> ()
                        n109 = call "OEE_PART_1.vi"("CYCLE TIME"=w525, "ACTUAL PROD TIME"=w526, "BREAKDOWN TOTAL TIME"=w527) -> ("Numeric"=→"IDEAL CYCLE TIME":i32, "CAPACITY"=w520:dbl, "ACTUAL TIME"=w511:i32)  [unwired: 5 in, 1 out]
                        "AVAILABLILITY TIME(MIN)" <- w511
                        "CAPACITY" <- w520
                        n110 = local read "Select Station"() -> (w513:string)
                        n111 = local read "Shift"() -> (w514:string)
                        n112 = call "OEE_PART_2_P.vi"("Refnum in"=w519, "Shift"=w514, "String"="ALL", "Select Station"=w513, "Form Date"=w523, "To Date"=w522, "AVAILABLILITY TIME"=w511, "CAPACITY"=w520) -> ("Refnum out"=w518:T2, "Array"=→"transposed array":string[][], "QUALITY"=→"QUALITY":dbl, "Production count"=→"Production count":i32, "OEE"=→"OEE":dbl, "PERFORMANCE"=→"PERFORMANCE":dbl)  [unwired: 2 in]
                        "Array" <- w527
                      }
                    }
                  }
                  frame "1" {
                    n113 = flat-sequence {
                      tunnel: w572 -> [w686]
                      tunnel: w571 -> [w684]
                      tunnel: [w670] -> w662
                      tunnel: [w685] -> w661
                      tunnel: w570 -> [_]
                      tunnel: [w689] -> w660
                      tunnel: [w669] -> w659
                      tunnel: [w668] -> w658
                      tunnel: [w666] -> w657
                      tunnel: w569 -> [w669]
                      tunnel: w568 -> [w668]
                      tunnel: ["Where BREAKDOWN_DATE between '%s'and '%s' and BREAKDOWN_STK_HOLD_ID ='%d' and  SHIFT_ID = '%d' "] -> w656
                      tunnel: [w666] -> w655
                      tunnel: w563 -> [w664]
                      tunnel: w662 -> [w750]
                      tunnel: w661 -> [w752]
                      tunnel: w660 -> [w747]
                      tunnel: w659 -> [w746]
                      tunnel: w658 -> [w745]
                      tunnel: [w749] -> w654
                      tunnel: [w751] -> w653
                      tunnel: [w747] -> w652
                      tunnel: [w737] -> w651
                      tunnel: [w743] -> w650
                      tunnel: [w746] -> w649
                      tunnel: [w745] -> w648
                      tunnel: w657 -> [w742]
                      tunnel: [w742] -> w647
                      tunnel: w656 -> [w739]
                      tunnel: [w739] -> w646
                      tunnel: [w738] -> w645
                      tunnel: w655 -> [w738]
                      tunnel: w563 -> [w736]
                      tunnel: [w736] -> w567
                      tunnel: w654 -> [w768]
                      tunnel: w653 -> [w766]
                      tunnel: w652 -> [w771]
                      tunnel: w651 -> [w770]
                      tunnel: w650 -> [w769]
                      tunnel: w649 -> [w763]
                      tunnel: w648 -> [w762]
                      tunnel: [w771] -> w644
                      tunnel: [w770] -> w643
                      tunnel: [w769] -> w642
                      tunnel: [w767] -> w641
                      tunnel: [w760] -> w640
                      tunnel: [w759] -> w639
                      tunnel: [w764] -> w638
                      tunnel: [w763] -> w637
                      tunnel: [w762] -> w636
                      tunnel: w647 -> [w758]
                      tunnel: [w758] -> w635
                      tunnel: w646 -> [w755]
                      tunnel: [w755] -> w634
                      tunnel: [w754] -> w633
                      tunnel: w645 -> [w754]
                      tunnel: w567 -> [w753]
                      tunnel: [w753] -> w566
                      tunnel: w644 -> [w792]
                      tunnel: w643 -> [w791]
                      tunnel: w642 -> [w790]
                      tunnel: w641 -> [w786]
                      tunnel: w640 -> [w789]
                      tunnel: w639 -> [w788]
                      tunnel: w638 -> [w784]
                      tunnel: w637 -> [w782]
                      tunnel: w636 -> [w781]
                      tunnel: [w792] -> w632
                      tunnel: [w791] -> w631
                      tunnel: [w790] -> w630
                      tunnel: [w789] -> w629
                      tunnel: [w788] -> w628
                      tunnel: [w785] -> w627
                      tunnel: [w779] -> w626
                      tunnel: [w778] -> w625
                      tunnel: [w783] -> w624
                      tunnel: [w782] -> w623
                      tunnel: [w781] -> w622
                      tunnel: w635 -> [w777]
                      tunnel: [w777] -> w621
                      tunnel: w634 -> [w774]
                      tunnel: [w774] -> w620
                      tunnel: [w773] -> w619
                      tunnel: w633 -> [w773]
                      tunnel: w566 -> [w772]
                      tunnel: [w772] -> w565
                      tunnel: w632 -> [w815]
                      tunnel: w631 -> [w814]
                      tunnel: w630 -> [w813]
                      tunnel: w629 -> [w812]
                      tunnel: w628 -> [w811]
                      tunnel: w627 -> [w807]
                      tunnel: w626 -> [w810]
                      tunnel: w625 -> [w809]
                      tunnel: w624 -> [w806]
                      tunnel: w623 -> [w803]
                      tunnel: w622 -> [w802]
                      tunnel: [w815] -> w618
                      tunnel: [w814] -> w617
                      tunnel: [w813] -> w616
                      tunnel: [w812] -> w615
                      tunnel: [w811] -> w614
                      tunnel: [w810] -> w613
                      tunnel: [w809] -> w612
                      tunnel: [w805] -> w611
                      tunnel: [w804] -> w610
                      tunnel: [w800] -> w609
                      tunnel: [w799] -> w608
                      tunnel: [w803] -> w607
                      tunnel: [w802] -> w606
                      tunnel: w621 -> [w798]
                      tunnel: [w798] -> w605
                      tunnel: w620 -> [w795]
                      tunnel: [w795] -> w604
                      tunnel: [w794] -> w603
                      tunnel: w619 -> [w794]
                      tunnel: w565 -> [w793]
                      tunnel: [w793] -> w564
                      tunnel: w618 -> [w840]
                      tunnel: w617 -> [w839]
                      tunnel: w616 -> [w838]
                      tunnel: w615 -> [w837]
                      tunnel: w614 -> [w836]
                      tunnel: w613 -> [w835]
                      tunnel: w612 -> [w834]
                      tunnel: w611 -> [w828]
                      tunnel: w610 -> [w830]
                      tunnel: w609 -> [w833]
                      tunnel: w608 -> [w832]
                      tunnel: w607 -> [w825]
                      tunnel: w606 -> [w826]
                      tunnel: [w840] -> w602
                      tunnel: [w839] -> w601
                      tunnel: [w838] -> w600
                      tunnel: [w837] -> w599
                      tunnel: [w836] -> w598
                      tunnel: [w835] -> w597
                      tunnel: [w834] -> w596
                      tunnel: [w833] -> w595
                      tunnel: [w832] -> w594
                      tunnel: [w829] -> w593
                      tunnel: [w827] -> w592
                      tunnel: [w823] -> w591
                      tunnel: [w821] -> w590
                      tunnel: w605 -> [w822]
                      tunnel: w604 -> [w818]
                      tunnel: [w817] -> w589
                      tunnel: w603 -> [w817]
                      tunnel: w564 -> [w816]
                      tunnel: w602 -> [w867]
                      tunnel: w601 -> [w860]
                      tunnel: w600 -> [w851]
                      tunnel: w599 -> [w859]
                      tunnel: w598 -> [w849]
                      tunnel: w597 -> [w858]
                      tunnel: w596 -> [w847]
                      tunnel: w595 -> [w857]
                      tunnel: w594 -> [w845]
                      tunnel: w593 -> [w881]
                      tunnel: w592 -> [w880]
                      tunnel: w591 -> [w856]
                      tunnel: w590 -> [w843]
                      tunnel: [w881] -> w588
                      tunnel: [w880] -> w587
                      tunnel: [w874] -> w586
                      tunnel: [w867] -> w585
                      tunnel: [w866] -> w584
                      tunnel: [w865] -> w583
                      tunnel: [w864] -> w582
                      tunnel: [w863] -> w581
                      tunnel: [w862] -> w580
                      tunnel: [w861] -> w579
                      tunnel: [w860] -> w578
                      tunnel: [w859] -> w577
                      tunnel: [w858] -> w576
                      tunnel: [w857] -> w575
                      tunnel: [w856] -> w574
                      tunnel: [w841] -> w573
                      tunnel: w589 -> [w841]
                      tunnel: [w901] -> w555
                      tunnel: [w887] -> w546
                      tunnel: w588 -> [w888]
                      tunnel: w587 -> [w901]
                      tunnel: w586 -> [w886]
                      tunnel: w585 -> [w899]
                      tunnel: w584 -> [w897]
                      tunnel: w583 -> [w895]
                      tunnel: w582 -> [w893]
                      tunnel: w581 -> [w891]
                      tunnel: w580 -> [w889]
                      tunnel: w579 -> [w882]
                      tunnel: w578 -> [w898]
                      tunnel: w577 -> [w896]
                      tunnel: w576 -> [w894]
                      tunnel: w575 -> [w892]
                      tunnel: w574 -> [w890]
                      tunnel: w573 -> [w885]
                      tunnel: [w882] -> w560
                      frame #0 {
                        w677 = "%Y-%m-%d" ("time format string (%c)")
                        n114 = Decimal String To Number(string=w664) -> (number=w663:i32)  [unwired: 2 in, 1 out]
                        n115 = property on="Table" class="Tbl (strict)"("Visible"=TRUE) -> ()  [unwired: 2 in, 2 out]
                        n116 = Format Date/Time String(time format string (%c)=w677, seconds (now)=w669) -> (date/time string=w678:string)  [unwired: 1 in]
                        n117 = Format Date/Time String(time format string (%c)=w677, seconds (now)=w668) -> (date/time string=w676:string)  [unwired: 1 in]
                        n118 = Format Into String(format string="Where BREAKDOWN_DATE between '%s' and '%s' and  SHIFT_ID = '%d'  ", w678, w676, w663) -> (resulting string=w675:string)  [unwired: 2 in, 1 out]
                        n119 = call <vilib>:"DB Tools Select Data.vi"("condition"=w675, "error in (no error)"=w684, "columns"=string[] ["BREAKDOWN_DATE"], "table"="STATION_1_LOG_HISTORY", "connection reference"=w686) -> ("error out"=w671:errorcluster, "data"=w674:variant[][], "connection reference out"=w685:T2)  [unwired: 1 in]
                        n120 = property on="Table 2" class="Tbl (strict)"("Visible"=FALSE) -> ()  [unwired: 2 in, 2 out]
                        n121 = xnode "Database Variant To Data"("database variant"=w674, "error in (no error)"=w671, "type"=string[][] [] ("Elements Found")) -> ("data"=w672:string[][], "error out"=w670:errorcluster)
                        n122 = Index Array(array=w672, index (col)=0 ("disabled index (col)")) -> (element=w680:string[])  [unwired: 1 in]
                        n123 = call "Search_1d_array_element.vi"("Count in"=string[] [] ("Elements Found"), "BD Date"=w680, "Elements Found in"=string[] [] ("Elements Found")) -> ("Elements Found out"=w666:string[])  [unwired: 4 in, 2 out]
                        n124 = Build Array(w666) -> (w690:string[][])
                        n125 = Transpose 2D Array(2D array=w690) -> (transposed array=w689:string[][])
                      }
                      frame #1 {
                        n126 = call "Stack_holderwise_total_bd_count_&_duration_2.vi"("Refnum in"=w752, "BREAKDOWN_STK_HOLD_ID"=1, "condition"=w739, "Form Date"=w746, "To Date"=w745, "error in (no error)"=w750, "Shift"=w736) -> ("Refnum out"=w751:T2, "Count out"=w744:string[], "appended array"=w741:dbl[], "error out"=w749:errorcluster)  [unwired: 5 in]
                        n127 = call "NUMERIC TO STRING.vi"("appended array"=w741) -> ("Array"=w740:string[])  [unwired: 4 in]
                        n128 = call "Insert_empty_element_with_zero.vi"("searched date"=w744, "fixed date"=w742) -> ("O/P"=w737:string[])  [unwired: 9 in]
                        n129 = call "Insert_empty_element_with_zero.vi"("searched date"=w740, "fixed date"=w742) -> ("O/P"=w743:string[])  [unwired: 9 in]
                      }
                      frame #2 {
                        n130 = call "Stack_holderwise_total_bd_count_&_duration_2.vi"("Refnum in"=w766, "BREAKDOWN_STK_HOLD_ID"=2, "condition"=w755, "Form Date"=w763, "To Date"=w762, "error in (no error)"=w768, "Shift"=w753) -> ("Refnum out"=w764:T2, "Count out"=w761:string[], "appended array"=w757:dbl[], "error out"=w767:errorcluster)  [unwired: 5 in]
                        n131 = call "Insert_empty_element_with_zero.vi"("searched date"=w761, "fixed date"=w758) -> ("O/P"=w760:string[])  [unwired: 9 in]
                        n132 = call "NUMERIC TO STRING.vi"("appended array"=w757) -> ("Array"=w756:string[])  [unwired: 4 in]
                        n133 = call "Insert_empty_element_with_zero.vi"("searched date"=w756, "fixed date"=w758) -> ("O/P"=w759:string[])  [unwired: 9 in]
                      }
                      frame #3 {
                        n134 = call "Stack_holderwise_total_bd_count_&_duration_2.vi"("Refnum in"=w784, "BREAKDOWN_STK_HOLD_ID"=3, "condition"=w774, "Form Date"=w782, "To Date"=w781, "error in (no error)"=w786, "Shift"=w772) -> ("Refnum out"=w783:T2, "Count out"=w780:string[], "appended array"=w776:dbl[], "error out"=w785:errorcluster)  [unwired: 5 in]
                        n135 = call "Insert_empty_element_with_zero.vi"("searched date"=w780, "fixed date"=w777) -> ("O/P"=w779:string[])  [unwired: 9 in]
                        n136 = call "NUMERIC TO STRING.vi"("appended array"=w776) -> ("Array"=w775:string[])  [unwired: 4 in]
                        n137 = call "Insert_empty_element_with_zero.vi"("searched date"=w775, "fixed date"=w777) -> ("O/P"=w778:string[])  [unwired: 9 in]
                      }
                      frame #4 {
                        n138 = call "Stack_holderwise_total_bd_count_&_duration_2.vi"("Refnum in"=w806, "BREAKDOWN_STK_HOLD_ID"=4, "condition"=w795, "Form Date"=w803, "To Date"=w802, "error in (no error)"=w807, "Shift"=w793) -> ("Refnum out"=w805:T2, "Count out"=w801:string[], "appended array"=w797:dbl[], "error out"=w804:errorcluster)  [unwired: 5 in]
                        n139 = call "Insert_empty_element_with_zero.vi"("searched date"=w801, "fixed date"=w798) -> ("O/P"=w800:string[])  [unwired: 9 in]
                        n140 = call "NUMERIC TO STRING.vi"("appended array"=w797) -> ("Array"=w796:string[])  [unwired: 4 in]
                        n141 = call "Insert_empty_element_with_zero.vi"("searched date"=w796, "fixed date"=w798) -> ("O/P"=w799:string[])  [unwired: 9 in]
                      }
                      frame #5 {
                        n142 = call "Stack_holderwise_total_bd_count_&_duration_2.vi"("Refnum in"=w828, "BREAKDOWN_STK_HOLD_ID"=5, "condition"=w818, "Form Date"=w825, "To Date"=w826, "error in (no error)"=w830, "Shift"=w816) -> ("Refnum out"=w827:T2, "Count out"=w824:string[], "appended array"=w820:dbl[], "error out"=w829:errorcluster)  [unwired: 5 in]
                        n143 = call "NUMERIC TO STRING.vi"("appended array"=w820) -> ("Array"=w819:string[])  [unwired: 4 in]
                        n144 = call "Insert_empty_element_with_zero.vi"("searched date"=w824, "fixed date"=w822) -> ("O/P"=w823:string[])  [unwired: 9 in]
                        n145 = call "Insert_empty_element_with_zero.vi"("searched date"=w819, "fixed date"=w822) -> ("O/P"=w821:string[])  [unwired: 9 in]
                      }
                      frame #6 {
                        n146 = call "String to numeric.vi"("Array"=w851) -> ("Array 2"=w850:dbl[])  [unwired: 4 in]
                        n147 = call "String to numeric.vi"("Array"=w849) -> ("Array 2"=w848:dbl[])  [unwired: 4 in]
                        n148 = call "String to numeric.vi"("Array"=w847) -> ("Array 2"=w846:dbl[])  [unwired: 4 in]
                        n149 = call "String to numeric.vi"("Array"=w845) -> ("Array 2"=w844:dbl[])  [unwired: 4 in]
                        n150 = call "String to numeric.vi"("Array"=w843) -> ("Array 2"=w842:dbl[])  [unwired: 4 in]
                        n151 = Decimal String To Number(string=w856) -> (number=w875:i32[])  [unwired: 2 in, 1 out]
                        n152 = Decimal String To Number(string=w857) -> (number=w876:i32[])  [unwired: 2 in, 1 out]
                        n153 = Decimal String To Number(string=w858) -> (number=w877:i32[])  [unwired: 2 in, 1 out]
                        n154 = Decimal String To Number(string=w859) -> (number=w878:i32[])  [unwired: 2 in, 1 out]
                        n155 = Decimal String To Number(string=w860) -> (number=w873:i32[])  [unwired: 2 in, 1 out]
                        n156 = Compound Arithmetic op=ADD(w850, w848, w846, w844, w842) -> (w853:dbl[])
                        n157 = Build Array(w851) -> (w872:string[][])
                        n158 = Build Array(w849) -> (w871:string[][])
                        n159 = Build Array(w847) -> (w870:string[][])
                        n160 = Build Array(w845) -> (w869:string[][])
                        n161 = Build Array(w843) -> (w868:string[][])
                        n162 = Number To Fractional String(number=w853, precision (6)=i16 2) -> (F-format string=w852:string[])  [unwired: 2 in]
                        n163 = Compound Arithmetic op=ADD(w875, w876, w877, w878, w873) -> (w879:i32[])
                        n164 = Transpose 2D Array(2D array=w872) -> (transposed array=w866:string[][])
                        n165 = Transpose 2D Array(2D array=w871) -> (transposed array=w865:string[][])
                        n166 = Transpose 2D Array(2D array=w870) -> (transposed array=w864:string[][])
                        n167 = Transpose 2D Array(2D array=w869) -> (transposed array=w863:string[][])
                        n168 = Transpose 2D Array(2D array=w868) -> (transposed array=w862:string[][])
                        n169 = Number To Decimal String(number=w879) -> (decimal integer string=w874:string[])  [unwired: 1 in]
                        n170 = Build Array(w852) -> (w855:string[][])
                        n171 = Transpose 2D Array(2D array=w855) -> (transposed array=w861:string[][])
                      }
                      frame #7 {
                        n172 = Insert Into Array(array=w899, index (col)=1 ("disabled index (col)"), new element #1=w898, new element #2=w897, new element #3=w896, new element #4=w895, new element #5=w894, new element #6=w893, new element #7=w892, new element #8=w891, new element #9=w890, new element #10=w889, new element #11=w886, new element #12=w882) -> (w884:string[][])  [unwired: 1 in]
                        n173 = call "flot graph for month n year.vi"("BD Date"=w885, "error in (no error)"=w888, "Count total"=w886) -> ("error out"=w887:errorcluster, "Run-Time Status"=w883:cluster{"Array 2":timestamp[], dbl[]})  [unwired: 7 in]
                        n174 = local write "Run-Time Status"(w883) -> ()
                        n175 = local write "Table"(w884) -> ()
                      }
                    }
                    n176 = call "OEE_PART_1.vi"("CYCLE TIME"=w561, "ACTUAL PROD TIME"=w562, "BREAKDOWN TOTAL TIME"=w560) -> ("Numeric"=w553:i32, "CAPACITY"=w552:dbl, "ACTUAL TIME"=w551:i32)  [unwired: 5 in, 1 out]
                    n177 = call "OEE_PART_2_P.vi"("Refnum in"=w555, "Shift"=w557, "String"="ALL", "Select Station"=w556, "Form Date"=w559, "To Date"=w558, "AVAILABLILITY TIME"=w551, "CAPACITY"=w552) -> ("Refnum out"=w547:T2, "QUALITY"=w550:dbl, "OEE"=w548:dbl, "PERFORMANCE"=w549:dbl)  [unwired: 2 in, 2 out]
                    n178 = local write "PERFORMANCE"(w549) -> ()
                    n179 = local write "QUALITY"(w550) -> ()
                    n180 = local write "OEE"(w548) -> ()
                    n181 = local write "AVAILABLILITY TIME(MIN)"(w551) -> ()
                    n182 = local write "IDEAL CYCLE TIME"(w553) -> ()
                    n183 = local write "CAPACITY"(w552) -> ()
                  }
                  frame "2" {
                    n184 = flat-sequence {
                      tunnel: w928 -> [w1042]
                      tunnel: w927 -> [w1040]
                      tunnel: [w1026] -> w1018
                      tunnel: [w1041] -> w1017
                      tunnel: w926 -> [_]
                      tunnel: [w1045] -> w1016
                      tunnel: [w1025] -> w1015
                      tunnel: [w1024] -> w1014
                      tunnel: [w1022] -> w1013
                      tunnel: w925 -> [w1025]
                      tunnel: w924 -> [w1024]
                      tunnel: ["Where BREAKDOWN_DATE between '%s'and '%s' and BREAKDOWN_STK_HOLD_ID ='%d' and  SHIFT_ID = '%d' "] -> w1012
                      tunnel: [w1022] -> w1011
                      tunnel: w919 -> [w1020]
                      tunnel: w1018 -> [w1106]
                      tunnel: w1017 -> [w1108]
                      tunnel: w1016 -> [w1103]
                      tunnel: w1015 -> [w1102]
                      tunnel: w1014 -> [w1101]
                      tunnel: [w1105] -> w1010
                      tunnel: [w1107] -> w1009
                      tunnel: [w1103] -> w1008
                      tunnel: [w1093] -> w1007
                      tunnel: [w1099] -> w1006
                      tunnel: [w1102] -> w1005
                      tunnel: [w1101] -> w1004
                      tunnel: w1013 -> [w1098]
                      tunnel: [w1098] -> w1003
                      tunnel: w1012 -> [w1095]
                      tunnel: [w1095] -> w1002
                      tunnel: [w1094] -> w1001
                      tunnel: w1011 -> [w1094]
                      tunnel: w919 -> [w1092]
                      tunnel: [w1092] -> w923
                      tunnel: w1010 -> [w1124]
                      tunnel: w1009 -> [w1122]
                      tunnel: w1008 -> [w1127]
                      tunnel: w1007 -> [w1126]
                      tunnel: w1006 -> [w1125]
                      tunnel: w1005 -> [w1119]
                      tunnel: w1004 -> [w1118]
                      tunnel: [w1127] -> w1000
                      tunnel: [w1126] -> w999
                      tunnel: [w1125] -> w998
                      tunnel: [w1123] -> w997
                      tunnel: [w1116] -> w996
                      tunnel: [w1115] -> w995
                      tunnel: [w1120] -> w994
                      tunnel: [w1119] -> w993
                      tunnel: [w1118] -> w992
                      tunnel: w1003 -> [w1114]
                      tunnel: [w1114] -> w991
                      tunnel: w1002 -> [w1111]
                      tunnel: [w1111] -> w990
                      tunnel: [w1110] -> w989
                      tunnel: w1001 -> [w1110]
                      tunnel: w923 -> [w1109]
